vi "Create Notifiers.vi"(8 "error in":errorcluster) -> (0 "error out":errorcluster, 3 "Notifiers":T1)   [LabVIEW 2015, in "Notifiers.lvlib"]
doc: "Creates notifiers for handshaking and closing processes"
uses:
  Notifiers.lvlib
  Notifiers.ctl
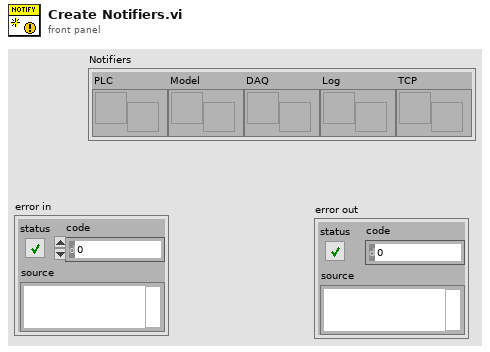
[diagram p1: front panel]
types:
  T1 = typedef "Notifiers.lvlib/Notifiers.ctl" = cluster{"PLC":refnum<notifier>, "Model":refnum<notifier>, "DAQ":refnum<notifier>, "Log":refnum<notifier>, "TCP":refnum<notifier>}
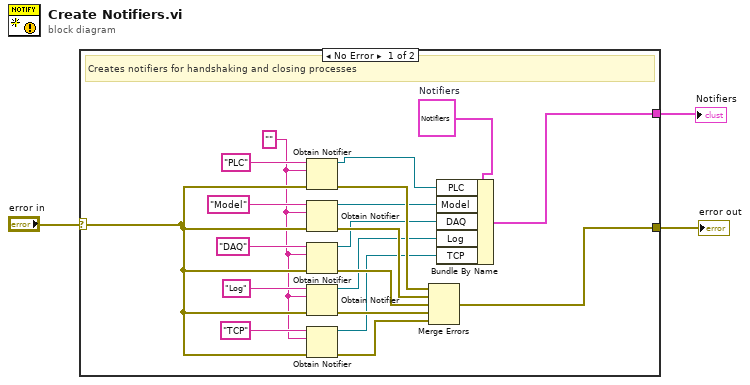
[diagram p0: block diagram]
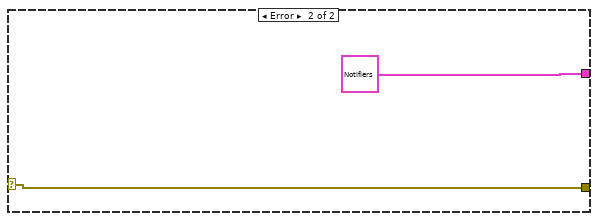
[diagram p2: hidden frame]
diagram:
  n1 = case shown="No Error" "error in" {
    selector: "error in" -> [w7 w25]
    tunnel: [w21 w25] -> w3
    tunnel: [w20 T1 {"PLC"=refnum, "Model"=refnum, "DAQ"=refnum, "Log"=refnum, "TCP"=refnum} ("Notifiers")] -> w2
    frame No Error {
      w6 = "" ("name (unnamed)")
      w4 = T1 {"PLC"=refnum, "Model"=refnum, "DAQ"=refnum, "Log"=refnum, "TCP"=refnum}  # Notifiers
      # "Creates notifiers for handshaking and closing processes"
      n2 = Obtain Notifier(name (unnamed)="PLC", notification data type=w6, error in (no error)=w7) -> (notifier out=w5:refnum<notifier>, error out=w22:errorcluster)  [unwired: 1 in, 1 out]
      n3 = Obtain Notifier(name (unnamed)="Model", notification data type=w6, error in (no error)=w7) -> (notifier out=w15:refnum<notifier>, error out=w19:errorcluster)  [unwired: 1 in, 1 out]
      n4 = Obtain Notifier(name (unnamed)="DAQ", notification data type=w6, error in (no error)=w7) -> (notifier out=w14:refnum<notifier>, error out=w16:errorcluster)  [unwired: 1 in, 1 out]
      n5 = Obtain Notifier(name (unnamed)="Log", notification data type=w6, error in (no error)=w7) -> (notifier out=w12:refnum<notifier>, error out=w11:errorcluster)  [unwired: 1 in, 1 out]
      n6 = Obtain Notifier(name (unnamed)="TCP", notification data type=w6, error in (no error)=w7) -> (notifier out=w9:refnum<notifier>, error out=w8:errorcluster)  [unwired: 1 in, 1 out]
      n7 = Merge Errors(w22, w19, w16, w11, w8) -> (w21:errorcluster)
      n8 = Bundle By Name(cluster=w4, "PLC"=w5, "Model"=w15, "DAQ"=w14, "Log"=w12, "TCP"=w9) -> (w20:T1)
    }
    frame Error {
    }
  }
  "error out" <- w3
  "Notifiers" <- w2
